vi "4-2 matrice 3xM - matrice max - matrice 100x ris1.vi"(0 "Numeric":dbl=4.0 format="%.2f") -> (1 "A(i)":dbl[](array[numeric])=[0.6258772987432666, 0.38667970942052454, 0.5446694698771044, 0.8956403572658223, 0.6109849714258033] format="%.2f", 2 "B(i)":dbl[](array[numeric]) format="%.2f")   [LabVIEW 2012]
panel:
  out "Array Constant 2":dbl[][](array[numeric]) format="%.2f"
  out "c(i)":dbl[][](array[numeric]) format="%.2f"
  out "b(i)":dbl[][](array[numeric]) format="%.2f"
  out "a(i)":dbl[][](array[numeric]) format="%.2f"
  out "Array Constant":dbl[][](array[numeric]) format="%.2f"
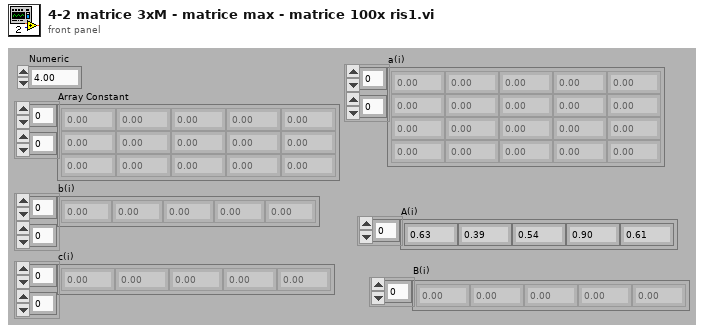
[diagram p1: front panel]
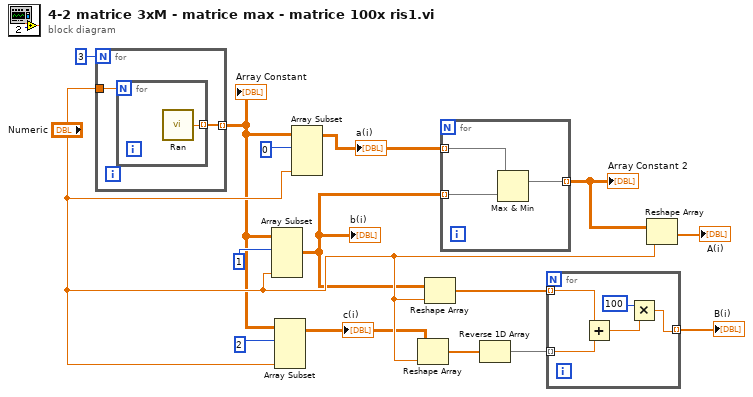
[diagram p0: block diagram]
diagram:
  n1 = for {
    N: 3 -> [_]
    tunnel: [w17] -> w2 mode=indexing
    tunnel: "Numeric" -> [w16]
    n2 = for {
      N: w16 -> [_]
      tunnel: [w18] -> w17 mode=indexing
      n3 = call "Ran.vi"() -> ("out num"=w18:dbl)  [unwired: 5 in]
    }
  }
  "Array Constant" <- w2
  n4 = Array Subset(array=w2, index (row)=1, length (col)="Numeric") -> (w7:dbl[][])  [unwired: 2 in]
  "b(i)" <- w7
  n5 = Array Subset(array=w2, index (row)=2, length (col)="Numeric") -> (w8:dbl[][])  [unwired: 2 in]
  "c(i)" <- w8
  n6 = Array Subset(array=w2, index (row)=0, length (col)="Numeric") -> (w12:dbl[][])  [unwired: 2 in]
  "a(i)" <- w12
  n7 = Reshape Array(w8, "Numeric") -> (w6:dbl[])
  n8 = Reshape Array(w7, "Numeric") -> (w4:dbl[])
  n9 = for {
    tunnel: w12 -> [w21] mode=indexing
    tunnel: w7 -> [w20] mode=indexing
    tunnel: [w19] -> w11 mode=indexing
    n10 = Max & Min(x=w21, y=w20) -> (max(x,y)=w19:dbl[])  [unwired: 1 out]
  }
  "Array Constant 2" <- w11
  n11 = Reverse 1D Array(array=w6) -> (reversed array=w5:dbl[])
  n12 = for {
    tunnel: w5 -> [w26] mode=indexing
    tunnel: w4 -> [w25] mode=indexing
    tunnel: [w22] -> w3 mode=indexing
    n13 = Add(x=w25, y=w26) -> (x+y=w23:dbl)
    n14 = Multiply(x=100, y=w23) -> (x*y=w22:dbl)
  }
  "B(i)" <- w3
  n15 = Reshape Array(w11, "Numeric") -> (→"A(i)":dbl[])
